vi "File_HandleSegmentation.vi"(8 "error in (no error)":errorcluster, 9 "Segment by":T1=enum."Size (MB)", 10 "Segment Every":dbl, 11 "File in":refnum<class "File.lvclass">) -> (0 "error out":errorcluster, 2 "Segment?":bool, 3 "File out":refnum<class "File.lvclass">)   [LabVIEW 2024, in "File.lvclass"]
doc: "Determine whether the segmentation conditions are met and if so, close the file and start a new TDMS file to log to (i.e. segment)."
uses:
  File.lvclass
  SegmentationOptions.ctl
  File.lvclass/File.ctl
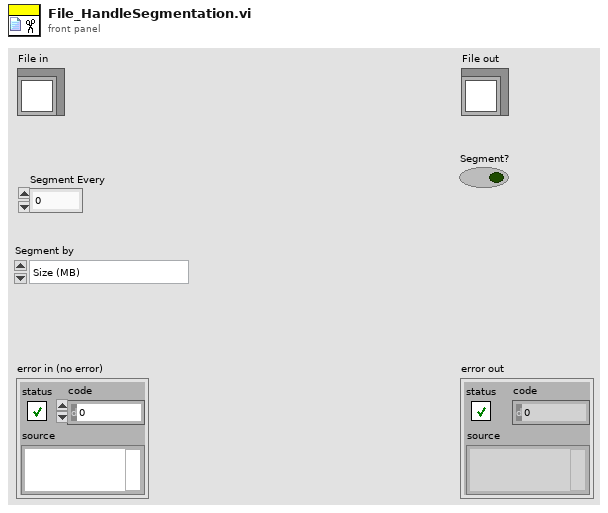
[diagram p1: front panel]
types:
  T1 = typedef "SegmentationOptions.ctl" = enum16{"Time (s)", "Size (MB)"}
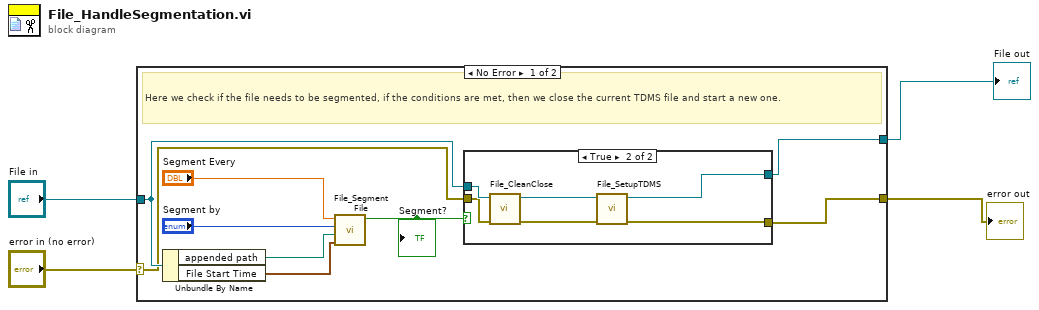
[diagram p0: block diagram]
diagram:
  n1 = case shown="No Error" "error in (no error)" {
    selector: "error in (no error)" -> [w9 w23]
    tunnel: [w10 w23] -> w3
    tunnel: [w11 w22] -> w1
    tunnel: "File in" -> [w12 w22]
    frame No Error {
      # "Here we check if the file needs to be segmented, if the conditions are met, then we close the current TDMS file and start a new one."
      n2 = Unbundle By Name(w12) -> ("appended path"=w6:path, "File Start Time"=w5:timestamp)
      n3 = call "File_Segment File.vi"("current time in"=w5, "path in"=w6, "Segment by"="Segment by", "Segment Every"="Segment Every") -> ("Boolean"=w13:bool)  [unwired: 7 in]
      "Segment?" <- w13
      n4 = case shown="True" w13 {
        tunnel: w9 -> [w14 w20]
        tunnel: w12 -> [w15 w21]
        tunnel: [w15 w17] -> w11
        tunnel: [w14 w16] -> w10
        frame False {
        }
        frame True {
          n5 = call-dynamic "File_CleanClose.vi"("error in (no error)"=w20, "File in"=w21) -> ("error out"=w18:errorcluster, "File out"=w19:refnum<class "File.lvclass">)  [unwired: 8 in]
          n6 = call-dynamic "File_SetupTDMS.vi"("error in (no error)"=w18, "File in"=w19) -> ("error out"=w16:errorcluster, "File out"=w17:refnum<class "File.lvclass">)  [unwired: 8 in]
        }
      }
    }
    frame Error {
    }
  }
  "error out" <- w3
  "File out" <- w1
